vi "Write Lockin Digitizer Configuration.vi"(8 "error in (no error)":errorcluster, 10 "Configuration":T1={"Post-trigger delay"=0.01, "Post-trigger duration"=0.1, "Rate"=1000000.0, "Ranges"=[10.0], "Re-name channels"=[], "Active channels"="0:1", "External\nclock"=FALSE, "Frequencies"=[], "Monitor time\nconstant"=1.0, "Output \namplitudes"=[], "Input\nchannles"=[], "Sync"=FALSE, "Lock-in input channel phases"=[]} {"Output \namplitudes" format="%#_6pV"; "Monitor time\nconstant" format="%#_6ps"; "Frequencies" format="%#_6pHz"; "Rate" format="%#_8pHz"; "Post-trigger duration" format="%#_6ps"; "Post-trigger delay" format="%#_6ps"; "Ranges" format="%#_6pV"}, 11 "DAQmx DAQmx Lockin Digitizer Driver in":refnum<class "DAQmx Lockin Digitizer Driver.lvclass">) -> (0 "error out":errorcluster, 3 "DAQmx DAQmx Lockin Digitizer Driver in":refnum<class "DAQmx Lockin Digitizer Driver.lvclass">)   [LabVIEW 2021, in "DAQmx Lockin Digitizer Driver.lvclass"]
uses:
  DAQmx Lockin Digitizer Driver.lvclass
  C:/GitHub/NHMFL_Core/Libraries/Instruments/Instrument Driver/Instrument Driver.lvclass
  Instruments/Pulse Driver/Lockin Digitizer Driver/Lockin Digitizer Configuration.ctl
  DAQmx Lockin Digitizer Driver.lvclass/DAQmx Lockin Digitizer Driver.ctl
panel:
  # "Pulse config"
  # "Lock-in config"
  # "#0\n\n#1"
  # "Monitor config"
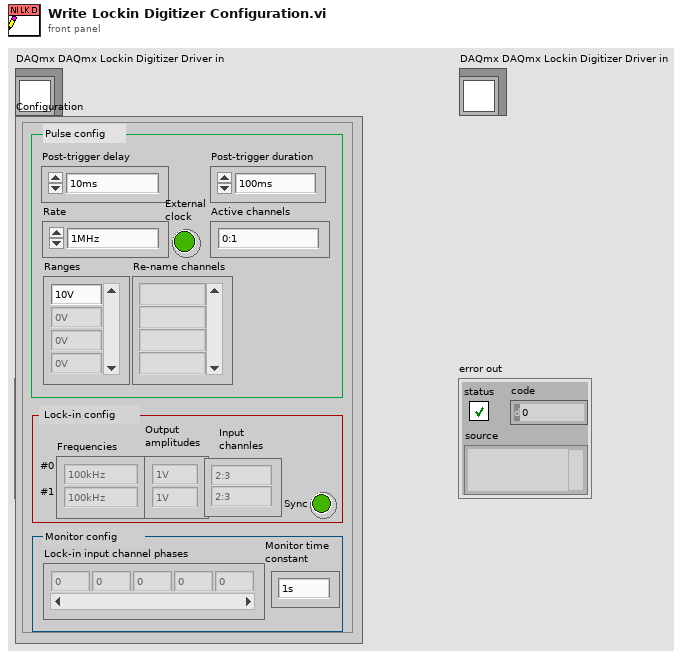
[diagram p1: front panel]
types:
  T1 = typedef "Lockin Digitizer Configuration.ctl" = cluster{"Post-trigger delay":dbl, "Post-trigger duration":dbl, "Rate":dbl, "Ranges":dbl[], "Re-name channels":string[], "Active channels":string, "External\nclock":bool, "Frequencies":dbl[], "Monitor time\nconstant":dbl, "Output \namplitudes":dbl[], "Input\nchannles":string[], "Sync":bool, "Lock-in input channel phases":dbl[]}
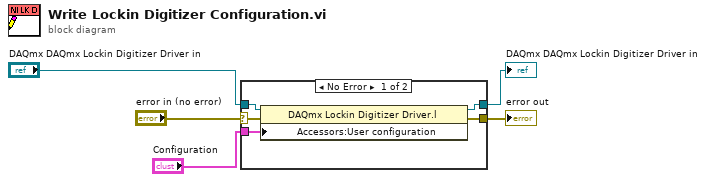
[diagram p0: block diagram]
diagram:
  n1 = case shown="No Error" "error in (no error)" {
    selector: "error in (no error)" -> [w10 w11]
    tunnel: [w9 w11] -> w1
    tunnel: [w7 w12] -> w2
    tunnel: "DAQmx DAQmx Lockin Digitizer Driver in" -> [w8 w12]
    tunnel: "Configuration" -> [w6 _]
    frame No Error {
      n2 = property class="DAQmx Lockin Digitizer Driver.l"(reference=w8, error in=w10, "Accessors:User configuration"=w6) -> (reference out=w7:refnum<class "DAQmx Lockin Digitizer Driver.lvclass">, error out=w9:errorcluster)
    }
    frame Error {
    }
  }
  "error out" <- w1
  "DAQmx DAQmx Lockin Digitizer Driver in" <- w2
